vi "joy_pc.vi"() -> ()   [LabVIEW 2017]
uses:
  <vilib>/Utility/inputDevices.llb/joystickAcquire.vi
  <vilib>/Utility/inputDevices.llb/closeJoystick.vi
panel:
  out "button info":T1
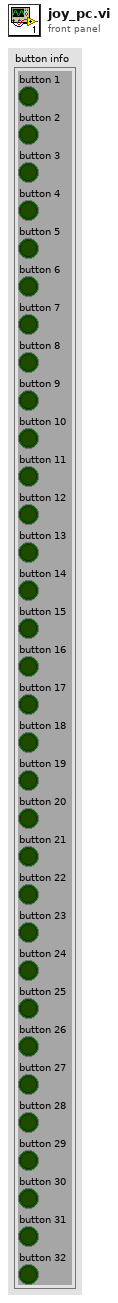
[diagram p1: front panel]
types:
  T1 = cluster{"button 1":bool, "button 2":bool, "button 3":bool, "button 4":bool, "button 5":bool, "button 6":bool, "button 7":bool, "button 8":bool, "button 9":bool, "button 10":bool, "button 11":bool, "button 12":bool, "button 13":bool, "button 14":bool, "button 15":bool, "button 16":bool, "button 17":bool, "button 18":bool, "button 19":bool, "button 20":bool, "button 21":bool, "button 22":bool, "button 23":bool, "button 24":bool, "button 25":bool, "button 26":bool, "button 27":bool, "button 28":bool, "button 29":bool, "button 30":bool, "button 31":bool, "button 32":bool}
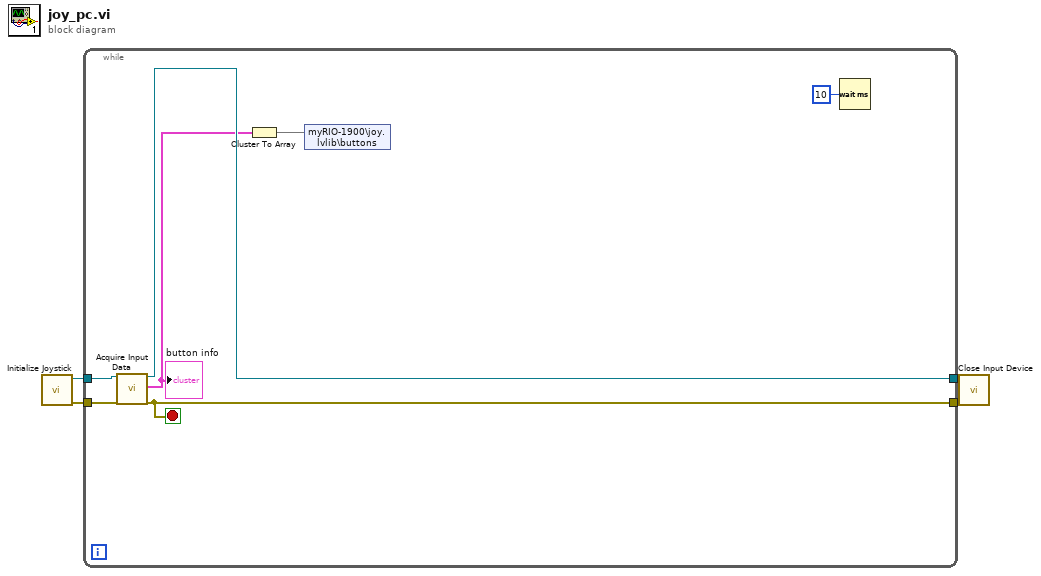
[diagram p0: block diagram]
diagram:
  n1 = call <vilib>:"Initialize Joystick.vi"() -> ("error out"=w4:errorcluster, "device ID"=w2:refnum<k1>)  [unwired: 10 in]
  n2 = while {
    tunnel: w4 -> [w11]
    tunnel: [w10] -> w3
    tunnel: w2 -> [w9]
    tunnel: [w8] -> w1
    stop <- w10 stop-if-true
    n3 = call-poly <vilib>:"Acquire Input Data.vi"("device ID"=w9, "error in (no error)"=w11) -> ("device ID"=w8:refnum<k1>, "button info"=w6:T1, "error out"=w10:errorcluster)  [unwired: 13 in, 2 out]
    "button info" <- w6
    n4 = Cluster To Array(cluster=w6) -> (array=w7:bool[])
    n5 = shared-variable "myRIO-1900\\joy.lvlib\\buttons"(w7) -> ()  [unwired: 1 in, 1 out]
    n6 = Wait (ms)(milliseconds to wait=u32 10) -> ()  [unwired: 1 out]
  }
  n7 = call-poly <vilib>:"Close Input Device.vi"("error in (no error)"=w3, "device ID"=w1) -> ()  [unwired: 8 in, 1 out]
